vi "IFilterPut.vi"(0 "PRIORLib.IFilterIn":refnum<k7>, 1 "Position":i16) -> (2 "PRIORLib.IFilterrOut":refnum<k7>, 3 "error out":errorcluster, 4 "Return":i32)   [LabVIEW 2016]
panel:
  in  "Filter Wheel #":i32=1
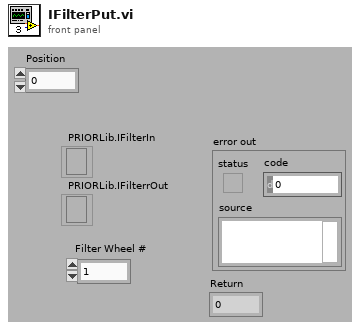
[diagram p1: front panel]
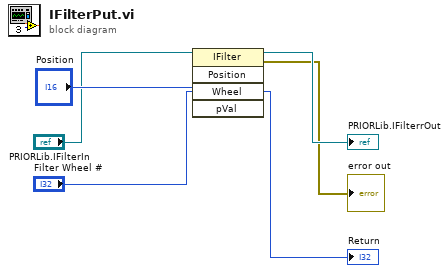
[diagram p0: block diagram]
diagram:
  n1 = invoke class="IFilter" method="Position"(reference="PRIORLib.IFilterIn", "Wheel"="Filter Wheel #", "pVal"="Position") -> (reference out=→"PRIORLib.IFilterrOut":refnum<k7>, error out=→"error out":errorcluster, "Wheel"=→"Return":i32)  [unwired: 2 in, 2 out]
